vi "SCMP - Run Cbk dwell time.vi"(8 "error in (no error)":errorcluster, 11 "Dwell time [s]":sgl format="%.2f") -> (0 "error out":errorcluster, 3 "Aborted?":bool)   [LabVIEW 2014]
doc: "Wait subVI for cbk command dwell time."
panel:
  in  "Abort Dwell Time":bool
  out "Time to end [s]":dbl format="%.1f"
  # "Cookbook command"
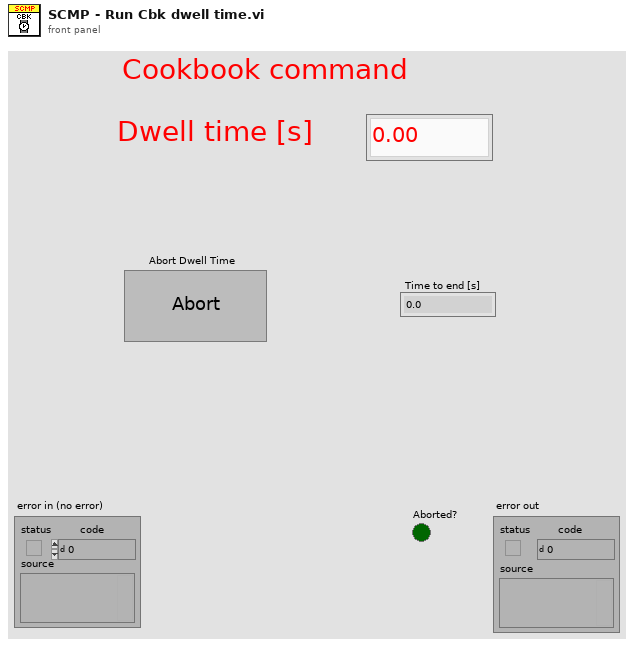
[diagram p1: front panel]
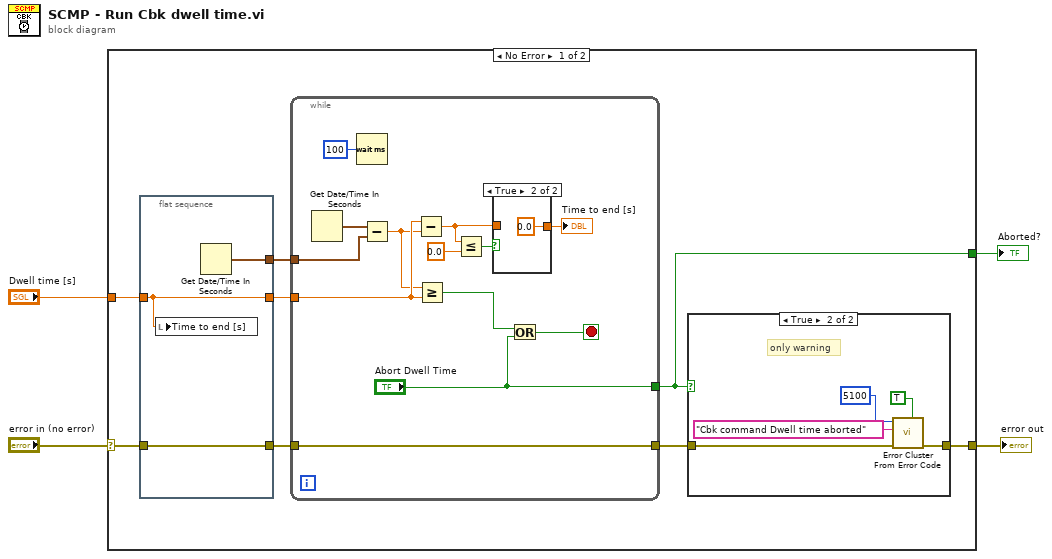
[diagram p0: block diagram]
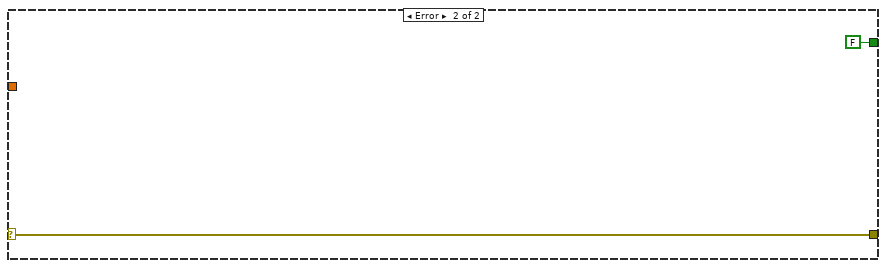
[diagram p4: hidden frame]
diagram:
  n1 = case shown="No Error" "error in (no error)" {
    selector: "error in (no error)" -> [w8 w38]
    tunnel: [w11 w38] -> w3
    tunnel: "Dwell time [s]" -> [w10 _]
    tunnel: [w5 FALSE ("Abort Dwell Time")] -> w1
    frame No Error {
      n2 = flat-sequence {
        tunnel: [w15] -> w12
        tunnel: w10 -> [w14]
        tunnel: [w14] -> w9
        tunnel: w8 -> [w13]
        tunnel: [w13] -> w7
        frame #0 {
          n3 = local write "Time to end [s]"(w14) -> ()
          n4 = Get Date/Time In Seconds() -> (seconds since 1Jan1904=w15:timestamp)
        }
      }
      n5 = while {
        tunnel: w12 -> [w32]
        tunnel: w9 -> [w28]
        tunnel: ["Abort Dwell Time"] -> w5
        tunnel: [w27] -> w6
        tunnel: w7 -> [w27]
        stop <- w30 stop-if-true
        n6 = Get Date/Time In Seconds() -> (seconds since 1Jan1904=w33:timestamp)
        n7 = Wait (ms)(milliseconds to wait=u32 100) -> ()  [unwired: 1 out]
        n8 = Subtract(x=w33, y=w32) -> (x-y=w26:dbl)
        n9 = Subtract(x=w28, y=w26) -> (x-y=w23:dbl)
        n10 = Greater Or Equal?(x=w26, y=w28) -> (x >= y?=w31:bool)
        n11 = Less Or Equal?(x=w23, y=0.0) -> (x <= y?=w24:bool)
        n12 = case shown="True" w24 {
          tunnel: [w35 0.0] -> w22
          tunnel: w23 -> [w35 _]
          frame False {
          }
          frame True {
          }
        }
        "Time to end [s]" <- w22
        n13 = Or(x=w31, y="Abort Dwell Time") -> (x .or. y?=w30:bool)
      }
      n14 = case shown="True" w5 {
        tunnel: [w16 w21] -> w11
        tunnel: w6 -> [w16 w19]
        frame False {
        }
        frame True {
          # "only warning"
          n15 = call <vilib>:"Error Cluster From Error Code.vi"("is warning? (False)"=TRUE ("show call chain? (False)"), "error in (no error)"=w19, "error message (\"\")"="Cbk command Dwell time aborted" ("error message (\"\")"), "error code (0)"=5100) -> ("error out"=w21:errorcluster)  [unwired: 5 in]
        }
      }
    }
    frame Error {
    }
  }
  "error out" <- w3
  "Aborted?" <- w1
